vi "Read Configuration Data.vi"(8 "error in":errorcluster) -> (0 "error out":errorcluster, 3 "Configuration Data":T1)   [LabVIEW 2020]
uses:
  Configuration Data.ctl
  controls/MHL Configuration.ctl
  Controller/Controller Configuration.ctl
  Boiler/Boiler Configuration.ctl
  Boiler System Globals.vi
  <vilib>/Utility/config.llb/NI_LVConfig.lvlib
  Boiler/Boiler.lvlib
  Controller/Controller.lvlib
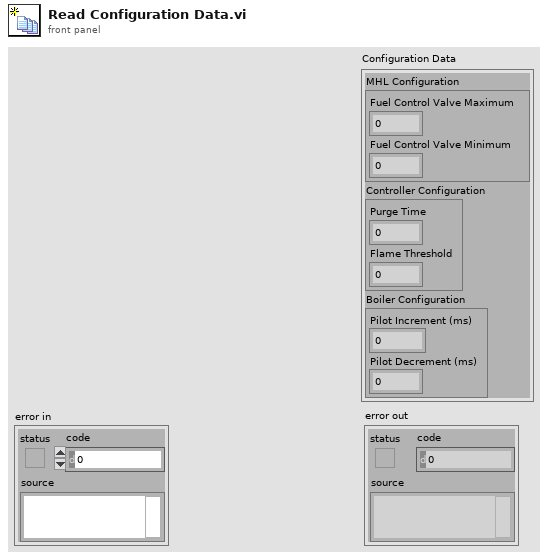
[diagram p1: front panel]
types:
  T1 = typedef "Configuration Data.ctl" = cluster{"MHL Configuration":T2, "Controller Configuration":T3, "Boiler Configuration":T4}
  T2 = typedef "MHL Configuration.ctl" = cluster{"Fuel Control Valve Maximum":dbl, "Fuel Control Valve Minimum":dbl}
  T3 = typedef "Controller.lvlib/Controller Configuration.ctl" = cluster{"Purge Time":u32, "Flame Threshold":u32}
  T4 = typedef "Boiler.lvlib/Boiler Configuration.ctl" = cluster{"Pilot Increment (ms)":u32, "Pilot Decrement (ms)":u32}
  T5 = enum32{"invalid app kind", "Development System", "Run Time System", "Student Edition", "Embedded LabVIEW", "Evaluation", "Custom"}
  T6 = typedef "NI_LVConfig.lvlib/Config Data RefNum.ctl" = refnum<k1>
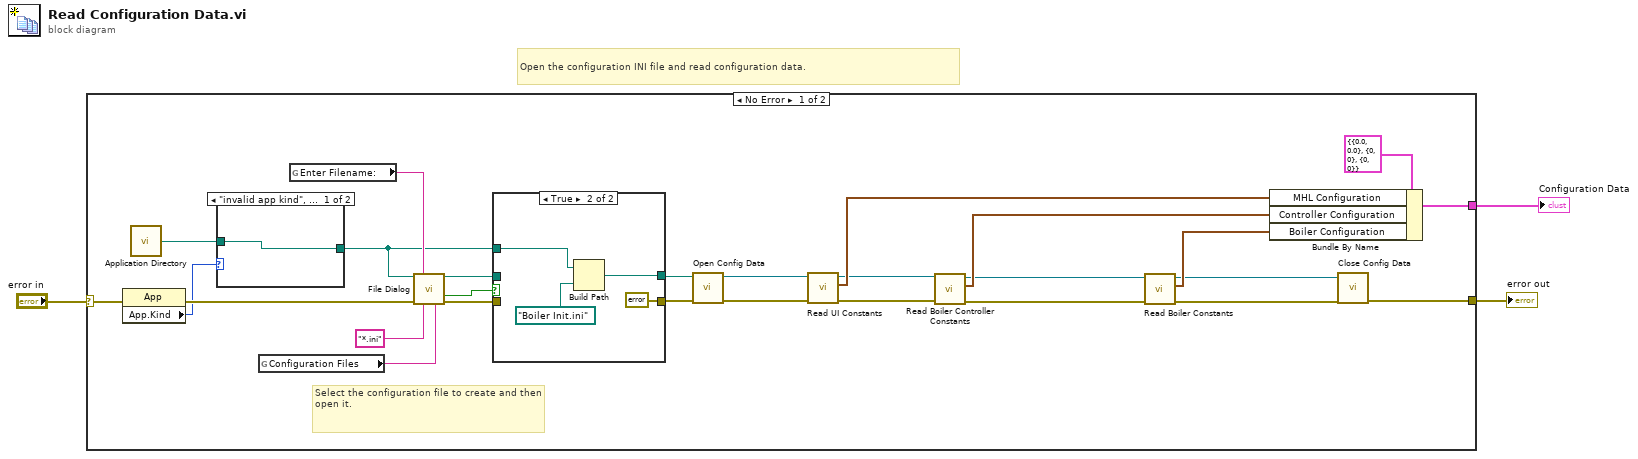
[diagram p0: block diagram]
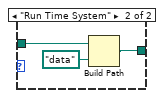
[diagram p2: hidden frame]
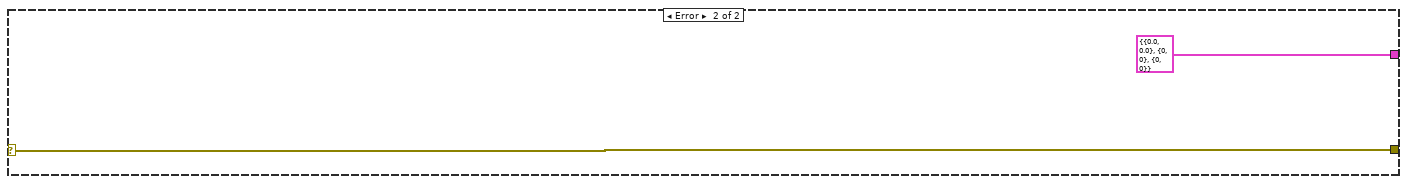
[diagram p4: hidden frame]
diagram:
  # "Open the configuration INI file and read configuration data."
  n1 = case shown="No Error" "error in" {
    selector: "error in" -> [w19 w42]
    tunnel: [w25 w42] -> w3
    tunnel: [w14 T1 {"MHL Configuration"={"Fuel Control Valve Maximum"=0.0, "Fuel Control Valve Minimum"=0.0}, "Controller Configuration"={"Purge Time"=0, "Flame Threshold"=0}, "Boiler Configuration"={"Pilot Increment (ms)"=0, "Pilot Decrement (ms)"=0}} ("Configuration Data")] -> w1
    frame No Error {
      # "Select the configuration file to create and then open it."
      n2 = property class="App"(error in=w19) -> (error out=w18:errorcluster, "App.Kind"=w17:T5)  [unwired: 1 in, 1 out]
      n3 = call <vilib>:"Application Directory.vi"() -> ("Application Directory"=w16:path)
      n4 = case shown="\"invalid app kind\", Default" w17 {
        tunnel: w16 -> [w31 w34]
        tunnel: [w31 w32] -> w15
        frame "invalid app kind", Default {
        }
        frame "Run Time System" {
          n5 = Build Path(base path=w34, name or relative path=path "data") -> (appended path=w32:path)
        }
      }
      n6 = global read "Boiler System Globals.vi" "Configuration Files"() -> (w28:string)
      n7 = global read "Boiler System Globals.vi" "Enter Filename:"() -> (w30:string)
      n8 = call "File Dialog"("start path"=w15, "prompt"=w30, "error in"=w18, "pattern (all files)"="*.ini", "pattern label"=w28) -> ("selected path"=w24:path, "cancelled"=w22:bool, "error out"=w21:errorcluster)  [unwired: 7 in, 1 out]
      n9 = case shown="True" w22 {
        tunnel: w15 -> [_ w39]
        tunnel: [w36 w37] -> w23
        tunnel: w24 -> [w36 _]
        tunnel: [w35 errorcluster {"status"=FALSE, "code"=0, "source"=""} ("error out")] -> w20
        tunnel: w21 -> [w35 _]
        frame False {
        }
        frame True {
          n10 = Build Path(base path=w39, name or relative path=path "Boiler Init.ini") -> (appended path=w37:path)
        }
      }
      n11 = call <vilib>:"Open Config Data.vi"("error in (no error)"=w20, "configuration file path"=w23) -> ("error out"=w26:errorcluster, "refnum"=w27:T6)  [unwired: 1 in, 7 out]
      n12 = call "Read UI Constants.vi"("error in"=w26, "CFG File Refnum in"=w27) -> ("error out"=w11:errorcluster, "MHL Configuration"=w12:T2, "CFG File Refnum out"=w9:T6)  [unwired: 7 in]
      n13 = call "Read Boiler Controller Constants.vi"("error in"=w11, "CFG File Refnum in"=w9) -> ("error out"=w5:errorcluster, "Controller Configuration"=w10:T3, "CFG File Refnum out"=w7:T6)  [unwired: 7 in]
      n14 = call "Read Boiler Constants.vi"("error in"=w5, "CFG File Refnum in"=w7) -> ("error out"=w4:errorcluster, "Boiler Configuration"=w8:T4, "CFG File Refnum out"=w6:T6)  [unwired: 7 in]
      n15 = Bundle By Name(cluster=T1 {"MHL Configuration"={"Fuel Control Valve Maximum"=0.0, "Fuel Control Valve Minimum"=0.0}, "Controller Configuration"={"Purge Time"=0, "Flame Threshold"=0}, "Boiler Configuration"={"Pilot Increment (ms)"=0, "Pilot Decrement (ms)"=0}} ("Configuration Data"), "MHL Configuration"=w12, "Controller Configuration"=w10, "Boiler Configuration"=w8) -> (w14:T1)
      n16 = call <vilib>:"Close Config Data.vi"("error in (no error)"=w4, "refnum"=w6) -> ("error out"=w25:errorcluster)  [unwired: 1 in, 8 out]
    }
    frame Error {
    }
  }
  "error out" <- w3
  "Configuration Data" <- w1
